vi "rowWrapPolicy.vi"(8 "Error In":errorcluster, 11 "QFormLayout In":refnum<class "QFormLayout.lvclass">) -> (0 "Error Out":errorcluster, 2 "Value":T1 items=["DontWrapRows", "WrapLongRows", "WrapAllRows"], 3 "QFormLayout Out":refnum<class "QFormLayout.lvclass">)   [LabVIEW 2014, in "QFormLayout.lvclass"]
doc: "LabVIEW-specific documentation is not yet available. See <b>http://doc.qt.io/qt-5/QFormLayout.html#rowWrapPolicy</b>"
uses:
  QFormLayout.lvclass
  RowWrapPolicy.ctl
  LQ Core/LQIdentity/LQIdentity.lvclass/LQIdentity.ctl
  LQ Core/LQ Core.lvlib
  LQ Core/LQIdentity/LQIdentity.lvclass
panel:
  # "Copyright (c) 2016 Sze Howe Koh\n\nThis Source Code Form is subject to the terms of the Mozilla Public\nLicense, v. 2.0. If a copy of the MPL was not distributed with this\nfile, You can obtain one at http://mozilla.org/MPL/2.0/."
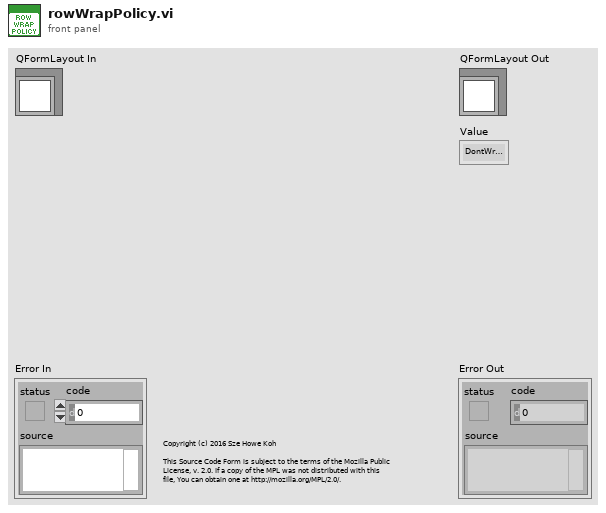
[diagram p1: front panel]
types:
  T1 = typedef "QFormLayout.lvclass/RowWrapPolicy.ctl" = i32
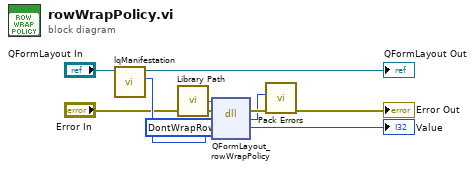
[diagram p0: block diagram]
diagram:
  w7 = T1 0 items=["DontWrapRows", "WrapLongRows", "WrapAllRows"] ("retVal")
  n1 = call "lqManifestation.vi"("LQIdentity in"="QFormLayout In") -> ("Manifestation"=w5:u64, "LQIdentity out"=→"QFormLayout Out":refnum<class "QFormLayout.lvclass">)  [unwired: 9 in]
  n2 = call "Library Path.vi"() -> ("Library Path"=w6:path)
  n3 = dll-call lib="?" fn="QFormLayout_rowWrapPolicy"(path in=w6, error in="Error In", "_retVal"=w7, "_instance"=w5) -> (error out=w3:errorcluster, w1:i32, "_retVal"=→"Value":i32)  [unwired: 2 in, 1 out]
  n4 = call "Pack Errors.vi"("Error In"=w3, "Error Code"=w1) -> ("Error Out"=→"Error Out":errorcluster)  [unwired: 9 in]
